vi "Write Magnetic Deviation.vi"(8 "error in (no error)":errorcluster, 10 "Magnetic Deviation":dbl, 11 "Compass Instrument in":refnum<class "Compass Instrument.lvclass">) -> (0 "error out":errorcluster, 3 "Compass Instrument out":refnum<class "Compass Instrument.lvclass">)   [LabVIEW 2015, in "Compass Instrument.lvlib" / "Compass Instrument.lvclass"]
uses:
  Compass Instrument.lvclass
  Compass Instrument.lvclass/Compass Instrument.ctl
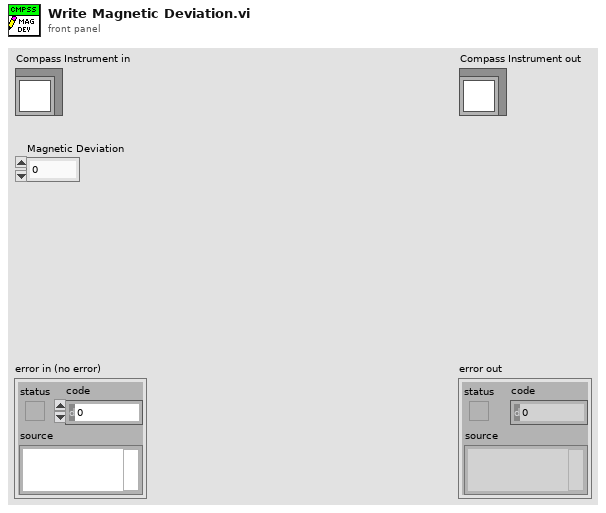
[diagram p1: front panel]
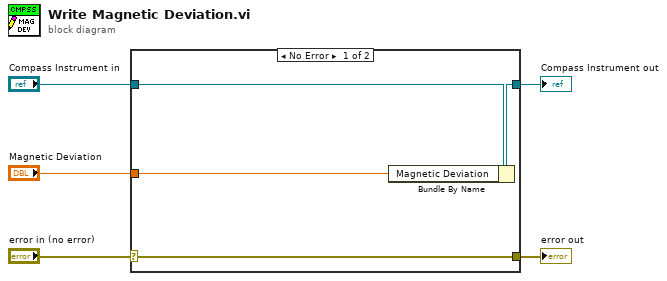
[diagram p0: block diagram]
diagram:
  n1 = case shown="No Error" "error in (no error)" {
    selector: "error in (no error)" -> [w9 w10]
    tunnel: [w9 w10] -> w4
    tunnel: [w7 w11] -> w2
    tunnel: "Compass Instrument in" -> [w8 w11]
    tunnel: "Magnetic Deviation" -> [w6 _]
    frame No Error {
      n2 = Bundle By Name(cluster=w8, "Magnetic Deviation"=w6) -> (w7:refnum<class "Compass Instrument.lvclass">)
    }
    frame Error {
    }
  }
  "error out" <- w4
  "Compass Instrument out" <- w2
